vi "Error Handler.vi"(1 "error In":errorcluster, 2 "ignore codes Array":i32[](array[numeric]), 3 "key":string) -> (0 "error Out":errorcluster)   [LabVIEW 2009, in "MoAgSy.lvlib" / "MoAgSy_Host.lvclass"]
doc: "<B>public</B> VI handels errors.\n<B>still in progress\nonly ask if error should be removed</B>\n\nF.Berck@gsi.de\nGSI Darmstadt 2009"
uses:
  MoAgSy_Host.lvclass
  <vilib>/Utility/error.llb/DialogType.ctl
  MoAgSy.lvlib
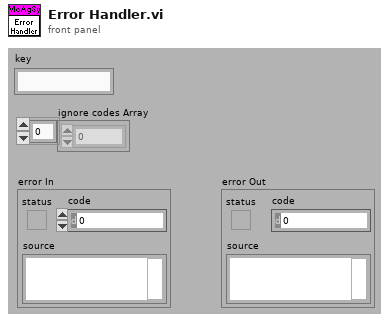
[diagram p1: front panel]
types:
  T1 = typedef "DialogType.ctl" = u16
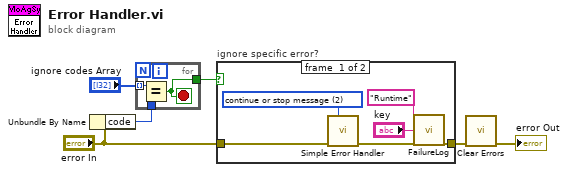
[diagram p0: block diagram]
diagram:
  n1 = Unbundle By Name("error In") -> ("code"=w3:i32)
  n2 = for {
    tunnel: w3 -> [w9]
    tunnel: "ignore codes Array" -> [w8] mode=indexing
    tunnel: [w7] -> w1
    stop <- w7 stop-if-true
    n3 = Equal?(x=w8, y=w9) -> (x = y?=w7:bool)
  }
  n4 = case "ignore specific error?" shown="False" w1 {
    tunnel: "error In" -> [w14 w16]
    tunnel: [w10 w16] -> w6
    frame #0 {
      w15 = T1 2 items=["no dialog", "OK message", "continue or stop message", "OK message + warnings", "continue/stop + warnings"] ("type of dialog (OK msg:1)")
      n5 = call <vilib>:"Simple Error Handler.vi"("type of dialog (OK msg:1)"=w15, "error in (no error)"=w14) -> ("error out"=w11:errorcluster)  [unwired: 3 in, 4 out]
      n6 = call "FailureLog.vi"("Section"="Runtime", "key"="key", "error in (no error)"=w11) -> ("error out"=w10:errorcluster)  [unwired: 16 in]
    }
    frame #1 {
    }
  }
  n7 = call <vilib>:"Clear Errors.vi"("error in (no error)"=w6) -> ("error out"=→"error Out":errorcluster)  [unwired: 6 in]
